vi "Meas Result Generate TWM InpZ Correction - Process Measurement.vi"(7 "table ref":refnum<vi>, 8 "error in":errorcluster, 10 "inpz unc config":T1, 11 "meas":T4={"swp cfg"={"N"=0, "R"=0, "f list"=[], "smpl delay"=0.0, "set delay"=0.0, "set delay np"=0.0, "meas root"=path "", "meas name"="", "meas a-index"=FALSE, "rnd sweep"=FALSE, "mode"=enum."Frequency", "swp mode"=enum."Linear", "avg"=0, "subrec"=0, "multi-freq"=FALSE, "selfcal"=FALSE, "selfcal period [h]"=0.0}, "bridge"={"type"=enum."TWM client", "TWM"={"pipe name"="", "parameters"=[], "handle"=0, "fixed aper [s]"=0.0, "f-list [Hz]"=[], "discrete f-list"=FALSE, "unc mode"=enum."None", "unc mcc"=0, "unc first"=FALSE, "alg id"=enum."TWM-LowZ - Low Z measurement"}, "last f"=0.0, "bias comp"={"bias type"=enum."dummy", "VISA"="", "Enable"=FALSE, "channel qu"=[], "channel Uinit"=[]}, "sim mode"=enum."Generic RLC network", "channel idns"=[], "sim phases"=1}, "src"={"type"=enum."Tektronix AFG3101C", "afg"={"VISA"="", "const"=0.0, "gen DC"=FALSE, "ext ref"=FALSE}, "cDAQ dds"={"device"="", "channels"=[], "mclk source"="", "mclk [Hz]"=0.0, "fs [Hz]"=0.0, "block [s]"=0.0, "buf [s]"=0.0, "task"="", "cmd queue"=refnum, "proc ref"=refnum, "smpl clock out"="/cDAQ3/PFI0", "export smpl clock"=FALSE, "DC ofs [V]"=[], "timebase source"="", "timebase mode"=enum."Local", "dither"=enum."Disabled", "dither level"=0.0, "phase [rad]"=[]}, "gain [V/A]"=1.0, "F5xxx session"={"VISA"="", "mode"=enum."AC voltage", "Earth on"=FALSE, "Ext ref lock"=FALSE}, "t3awg"={"VISA"="", "use ext ref"=FALSE, "ext ref [Hz]"=0.0, "load Z"=enum."High Z", "ramdac max n"=0, "noise dither [V]"=0.0, "t3awg fs rules"=[], "channels"=0, "ramdac min n"=0}}, "results"=refnum, "dvm"={"type"=enum."Disabled", "F5790"={"VISA"="", "Input"=enum."input 1", "Digital filter restart"=enum."medium", "hi resolution"=enum."off", "Digital filter mode"=enum."off", "ext guard"=FALSE}}, "thermo"={"type"=enum."COMET Tx5xx (ethernet)", "comment"="", "tag"="", "refresh"=5.0, "IP"="", "port"=502, "VISA"="", "last readout"=timestamp(0 s since 1904-01-01), "TCP ref"=refnum, "VISA sess"="", "idn"="", "press"=0.0, "RH"=0.0, "temp"=0.0, "pres cor"=[], "RH cor"=[], "temp cor"=[], "try left"=0, "failed"=FALSE, "RTD set"=[], "RTD inv"=[], "range"=0.0, "net mode"=enum."MODBUS", "try fail"=enum."Stop trying - return NaN", "timeout [s]"=0.0, "max retries"=0, "sim t [deg]"=0.0, "status"=0}} {"thermo"."status" items=["ok", "retry", "failed"]; "thermo"."RTD inv" format="%.1f"; "thermo"."RTD set" format="%.1f"; "thermo"."temp cor" format="%.1f"; "thermo"."RH cor" format="%.1f"; "thermo"."pres cor" format="%.1f"; "thermo"."refresh" min=0.1 max=1000.0 format="%.2f"; "src"."t3awg"."t3awg fs rules"."fs-step [Hz]" format="%#_6p"; "src"."t3awg"."t3awg fs rules"."fs-max [Hz]" format="%#_6p"; "src"."t3awg"."t3awg fs rules"."for f0 <" format="%#_6p"; "src"."t3awg"."t3awg fs rules"."fs-min [Hz]" format="%#_6p"; "src"."cDAQ dds"."channels" min=0 step=1; "bridge"."TWM"."f-list [Hz]" format="%#_6p"; "swp cfg"."f list"."bias" format="%#_3p"; "swp cfg"."f list"."level" format="%#_3p"; "swp cfg"."f list"."fs [Hz]" format="%#_5p"; "swp cfg"."f list"."time [s]" format="%#_3p"; "swp cfg"."f list"."f/fs" format="%#_3p"; "swp cfg"."f list"."periods" format="%#_3f"; "swp cfg"."f list"."f [Hz]" format="%#_5p"}) -> (0 "error out":errorcluster, 3 "correction data":T2)   [LabVIEW 2020]
doc: "Generates input impedance correction matrix for TWM."
uses:
  meas session.ctl
  Meas Sweep Config.ctl
  Meas Freq Info.ctl
  meas_swp_mode.ctl
  meas_sweep_flist_mode.ctl
  bridge/Bridge Session.ctl
  bridge/Bridge Type.ctl
  drivers/TWM client/TWM Session.ctl
  drivers/TWM client/TWM parameters.ctl
  drivers/TWM client/Meas Proc QWTB Uncertainty Mode.ctl
  bridge/Bridge Algorithm.ctl
  bridge/Bridge Bias Session.ctl
  bridge/Bridge Bias Type.ctl
  bridge/Bridge Sim Mode.ctl
  source/Source Session.ctl
  source/Source Type.ctl
  drivers/AFG3101C/AFG3101C Session.ctl
  drivers/cDAQ DDS/cDAQ DDS Session.ctl
  drivers/cDAQ DDS/cDAQ DDS Setup.ctl
  drivers/cDAQ DDS/cDAQ DDS Timebase Mode.ctl
  drivers/cDAQ DDS/cDAQ DDS Dither.ctl
  drivers/Fluke 5XXX/top_lev/F5xxx_session.ctl
  drivers/Fluke 5XXX/top_lev/F5xxx_output_mode.ctl
  drivers/T3AWG3K/toplevel/T3AWG Session.ctl
  drivers/T3AWG3K/toplevel/T3AWG Load Z.ctl
  drivers/T3AWG3K/toplevel/fgen_ramdac_fs_rules.ctl
  results/Meas Results Ref.ctl
  results/Meas Results.ctl
  bridge/Bridge Frequency Readings Data.ctl
  drivers/TWM client/Meas Proc QWTB Spectrum Data.ctl
  drivers/TWM client/TWM Phase Info.ctl
  dvm/dvm session.ctl
  dvm/dvm type.ctl
  drivers/Fluke 5790A/top_level/F5790 session.ctl
  thermo/thermo.ctl
  thermo/thermo_types.ctl
  thermo/Thermometer Fail Action.ctl
  Meas Results TWM Digitizer Correction Data.ctl
  results/Meas Results Correction Structuring Mode.ctl
  Meas Results TWM InpZ Correction Uncertainty Config.ctl
  results/Meas Results Sweep Data Uncertainty Mode.ctl
  results/Impedance Equivalent Circuit.ctl
  drivers/T3AWG3K/Active Technologies AWG3000.lvlib
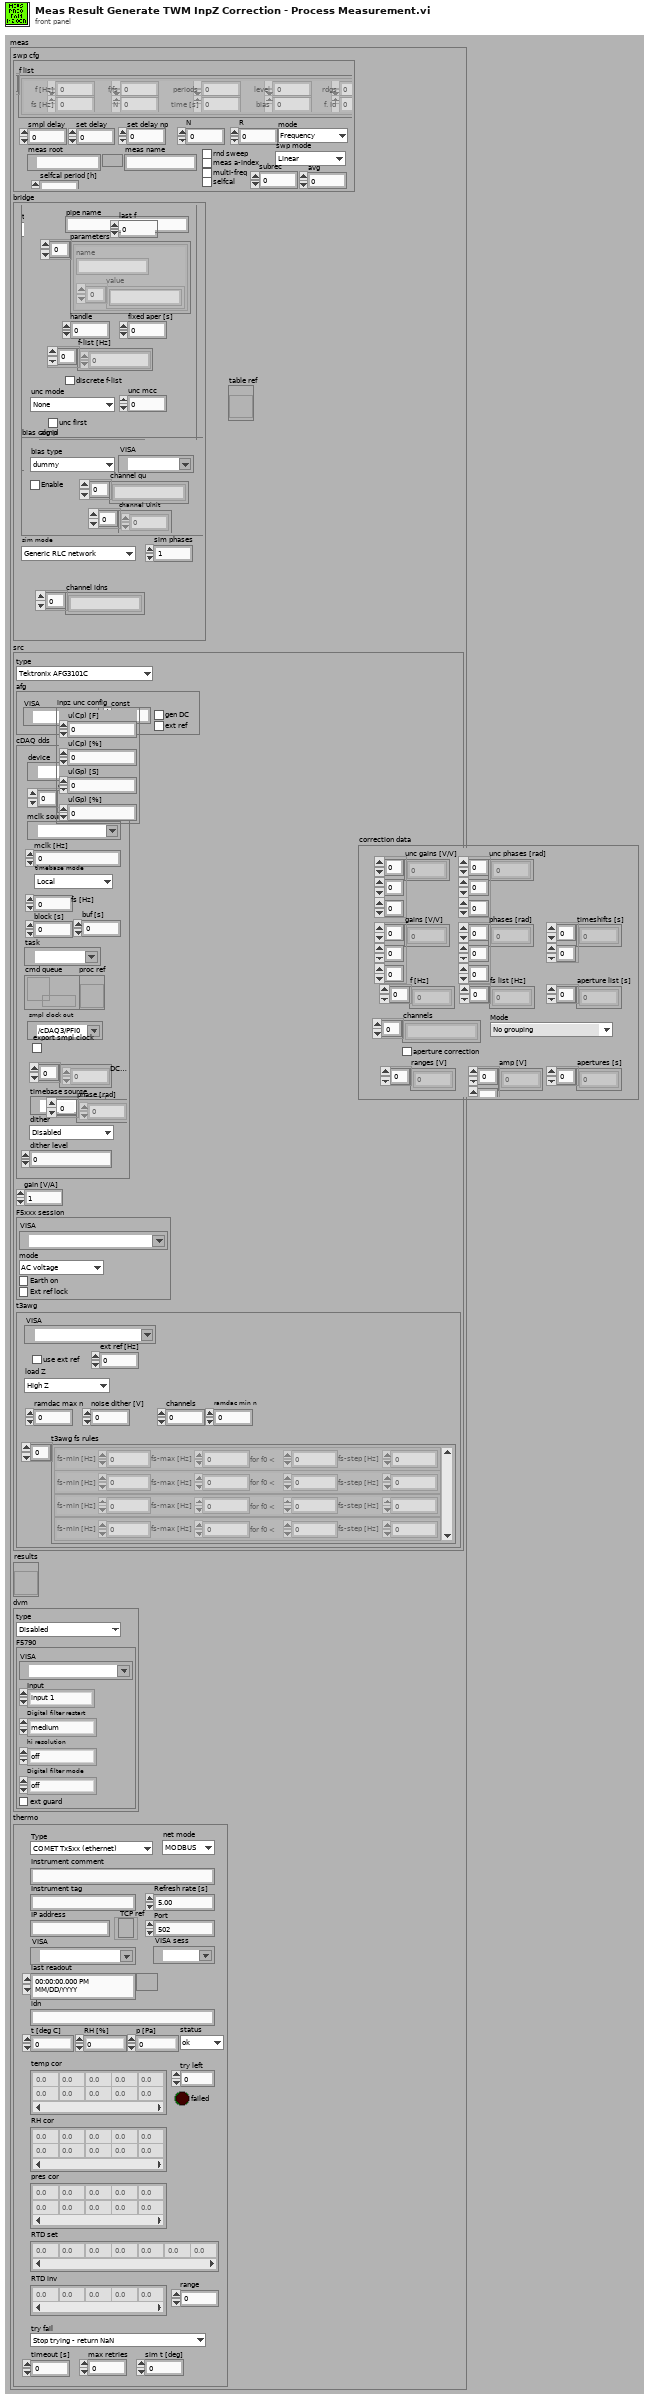
[diagram p1: front panel]
types:
  T1 = typedef "Meas Results TWM InpZ Correction Uncertainty Config.ctl" = cluster{"u(Cp) [F]":dbl, "u(Cp) [%]":dbl, "u(Gp) [S]":dbl, "u(Gp) [%]":dbl}
  T2 = typedef "Meas Results TWM Digitizer Correction Data.ctl" = cluster{"gains [V/V]":dbl[][][], "phases [rad]":dbl[][][], "timeshifts [s]":dbl[][], "f [Hz]":dbl[], "fs list [Hz]":dbl[], "aperture list [s]":dbl[], "channels":string[], "Mode":T3, "aperture correction":bool, "ranges [V]":dbl[], "amp [V]":dbl[][], "apertures [s]":dbl[], "unc gains [V/V]":dbl[][][], "unc phases [rad]":dbl[][][]}
  T3 = typedef "Meas Results Correction Structuring Mode.ctl" = enum16{"No grouping", "Group by apertures (3458A)", "Group by fs (generic digitizer)"}
  T4 = typedef "meas session.ctl" = cluster{"swp cfg":T5, "bridge":T9, "src":T18, "results":T29, "dvm":T30, "thermo":T33}
  T5 = typedef "Meas Sweep Config.ctl" = cluster{"N":i32, "R":i32, "f list":T6[], "smpl delay":dbl, "set delay":dbl, "set delay np":dbl, "meas root":path, "meas name":string, "meas a-index":bool, "rnd sweep":bool, "mode":T7, "swp mode":T8, "avg":i32, "subrec":i32, "multi-freq":bool, "selfcal":bool, "selfcal period [h]":dbl}
  T6 = typedef "Meas Freq Info.ctl" = cluster{"f [Hz]":dbl, "periods":dbl, "f/fs":dbl, "time [s]":dbl, "fs [Hz]":dbl, "N":i32, "level":dbl, "bias":dbl, "rdgs":i32, "f. id":i32}
  T7 = typedef "meas_swp_mode.ctl" = enum16{"Frequency", "Level", "Bias"}
  T8 = typedef "meas_sweep_flist_mode.ctl" = enum16{"Linear", "Log10"}
  T9 = typedef "Bridge Session.ctl" = cluster{"type":T10, "TWM":T11, "last f":dbl, "bias comp":T15, "sim mode":T17, "channel idns":string[], "sim phases":i32}
  T10 = typedef "Bridge Type.ctl" = enum16{"TWM client", "dummy"}
  T11 = typedef "TWM Session.ctl" = cluster{"pipe name":string, "parameters":T12[], "handle":i32, "fixed aper [s]":dbl, "f-list [Hz]":dbl[], "discrete f-list":bool, "unc mode":T13, "unc mcc":i32, "unc first":bool, "alg id":T14}
  T12 = typedef "TWM parameters.ctl" = cluster{"name":string, "value":string[]}
  T13 = typedef "Meas Proc QWTB Uncertainty Mode.ctl" = enum16{"None", "GUF", "Monte Carlo"}
  T14 = typedef "Bridge Algorithm.ctl" = enum16{"TWM-LowZ - Low Z measurement", "TWM-InpZ - Digitizer input Z measurement", "TWM-TIAZ - High Z using TIA"}
  T15 = typedef "Bridge Bias Session.ctl" = cluster{"bias type":T16, "VISA":refnum<visa-resource-name>, "Enable":bool, "channel qu":string[], "channel Uinit":dbl[]}
  T16 = typedef "Bridge Bias Type.ctl" = enum16{"dummy", "CMI LiBbias V1.0"}
  T17 = typedef "Bridge Sim Mode.ctl" = enum16{"Generic RLC network", "Interchannel transfer", "Input impedance"}
  T18 = typedef "Source Session.ctl" = cluster{"type":T19, "afg":T20, "cDAQ dds":T21, "gain [V/A]":dbl, "F5xxx session":T24, "t3awg":T26}
  T19 = typedef "Source Type.ctl" = enum16{"Tektronix AFG3101C", "cDAQ DAC", "Fluke 5xxx", "Agilent 33120A", "R&S SMT", "Teledyne LeCroy T3AWG", "dummy"}
  T20 = typedef "AFG3101C Session.ctl" = cluster{"VISA":refnum<visa-resource-name>, "const":dbl, "gen DC":bool, "ext ref":bool}
  T21 = typedef "cDAQ DDS Session.ctl" = cluster{"device":tag, "channels":i32[], "mclk source":tag, "mclk [Hz]":dbl, "fs [Hz]":dbl, "block [s]":dbl, "buf [s]":dbl, "task":refnum<k21>, "cmd queue":refnum<queue>, "proc ref":refnum<vi>, "smpl clock out":tag, "export smpl clock":bool, "DC ofs [V]":dbl[], "timebase source":tag, "timebase mode":T22, "dither":T23, "dither level":dbl, "phase [rad]":dbl[]}
  T22 = typedef "cDAQ DDS Timebase Mode.ctl" = enum16{"Local", "Take from ADC (e.g. NI 9238)", "Other source"}
  T23 = typedef "cDAQ DDS Dither.ctl" = enum16{"Disabled", "Gaussian"}
  T24 = typedef "F5xxx_session.ctl" = cluster{"VISA":refnum<visa-resource-name>, "mode":T25, "Earth on":bool, "Ext ref lock":bool}
  T25 = typedef "F5xxx_output_mode.ctl" = enum16{"AC voltage", "AC current"}
  T26 = typedef "Active Technologies AWG3000.lvlib/T3AWG Session.ctl" = cluster{"VISA":refnum<visa-resource-name>, "use ext ref":bool, "ext ref [Hz]":dbl, "load Z":T27, "ramdac max n":i32, "noise dither [V]":dbl, "t3awg fs rules":T28[], "channels":i32, "ramdac min n":i32}
  T27 = typedef "Active Technologies AWG3000.lvlib/T3AWG Load Z.ctl" = enum16{"High Z", "50 Ohm"}
  T28 = typedef "Active Technologies AWG3000.lvlib/fgen_ramdac_fs_rules.ctl" = cluster{"fs-min [Hz]":dbl, "fs-max [Hz]":dbl, "for f0 < ":dbl, "fs-step [Hz]":dbl}
  T29 = typedef "Meas Results Ref.ctl" = refnum<vi>
  T30 = typedef "dvm session.ctl" = cluster{"type":T31, "F5790":T32}
  T31 = typedef "dvm type.ctl" = enum16{"Disabled", "Simulated", "Fluke 5790A"}
  T32 = typedef "F5790 session.ctl" = cluster{"VISA":refnum<visa-resource-name>, "Input":enum16{"input 1", "input 2", "wide-band"}, "Digital filter restart":enum16{"medium", "fine", "coarse"}, "hi resolution":enum16{"off", "on"}, "Digital filter mode":enum16{"off", "fast", "medium", "slow"}, "ext guard":bool}
  T33 = typedef "thermo.ctl" = cluster{"type":T34, "comment":string, "tag":string, "refresh":dbl, "IP":string, "port":u16, "VISA":refnum<visa-resource-name>, "last readout":timestamp, "TCP ref":refnum<k5>, "VISA sess":refnum<visa-resource-name>, "idn":string, "press":dbl, "RH":dbl, "temp":dbl, "pres cor":dbl[][], "RH cor":dbl[][], "temp cor":dbl[][], "try left":i32, "failed":bool, "RTD set":dbl[], "RTD inv":dbl[], "range":dbl, "net mode":enum16{"MODBUS", "HTTP"}, "try fail":T35, "timeout [s]":dbl, "max retries":i32, "sim t [deg]":dbl, "status":u16}
  T34 = typedef "thermo_types.ctl" = enum16{"Disabled", "Simulated", "COMET Tx5xx (ethernet)", "Keithley 2002 (GPIB) + RTD", "Agilent 344xx (GPIB) + RTD"}
  T35 = typedef "Thermometer Fail Action.ctl" = enum16{"Stop trying - keep last value", "Stop trying - return NaN", "Generate error - stop sweep"}
  T36 = typedef "Meas Results Sweep Data Uncertainty Mode.ctl" = enum16{"ua(y)", "ua(y) (p=95%)", "uc(y) (p=95%)"}
  T37 = typedef "Meas Results.ctl" = cluster{"freqs":T38[][], "locked":bool, "last fid":i32, "modified":bool, "mjr name":string, "mnr name":string, "last spectra":T39[][], "saved?":bool, "TWM phase":T40[], "time start":timestamp, "time stop":timestamp, "equ cct":string}
  T38 = typedef "Bridge Frequency Readings Data.ctl" = cluster{"Udut":dbl[], "Iref":dbl[], "Udc":dbl[], "Idc":dbl[], "mjr":dbl[], "mnr":dbl[], "mjr_sh":dbl[], "mnr_sh":dbl[], "u(mjr)":dbl[], "u(mnr)":dbl[], "ua2(mjr)":dbl[], "ua2(mnr)":dbl[], "n":i32, "f [Hz]":dbl, "fs [Hz]":dbl, "aperture [s]":dbl, "Udvm":dbl[], "u(Udvm) [V]":dbl, "t_dut [degC]":dbl[], "RH_dut [%]":dbl[], "p_dut [Pa]":dbl[], "timestamp":timestamp[]}
  T39 = typedef "Meas Proc QWTB Spectrum Data.ctl" = cluster{"x":sgl[], "y":sgl[], "label":string}
  T40 = typedef "TWM Phase Info.ctl" = cluster{"ref chn id (I)":string, "dut chn id (U)":string, "ref chn range [V]":dbl, "dut chn range [V]":dbl, "aperture [s]":dbl, "fs [Hz]":dbl, "ref chn transducer (I)":string, "dut chn transducer (U)":string}
  T41 = typedef "Impedance Equivalent Circuit.ctl" = enum16{"Keep original", "Rs-Xs", "Gp-Bp", "Z-phid", "Z-phir", "Y-phid", "Y-phir", "Cp-D", "Cp-Q", "Cp-Rp", "Cp-Gp", "Cs-D", "Cs-Q", "Cs-Rs", "Ls-Rs", "Ls-Q", "Rs-Tau"}
  T42 = typedef "Meas Results Sweep Data.ctl" = cluster{"Udut":dbl[], "Iref":dbl[], "Udc":dbl[], "Idc":dbl[], "mjr":dbl[], "mnr":dbl[], "mjr_sh":dbl[], "mnr_sh":dbl[], "f [Hz]":dbl[], "n [-]":i32[], "fs [Hz]":dbl[], "aperture [s]":dbl[], "Udvm":dbl[], "t_dut [degC]":dbl[], "RH_dut [%]":dbl[], "p_dut [Pa]":dbl[]}
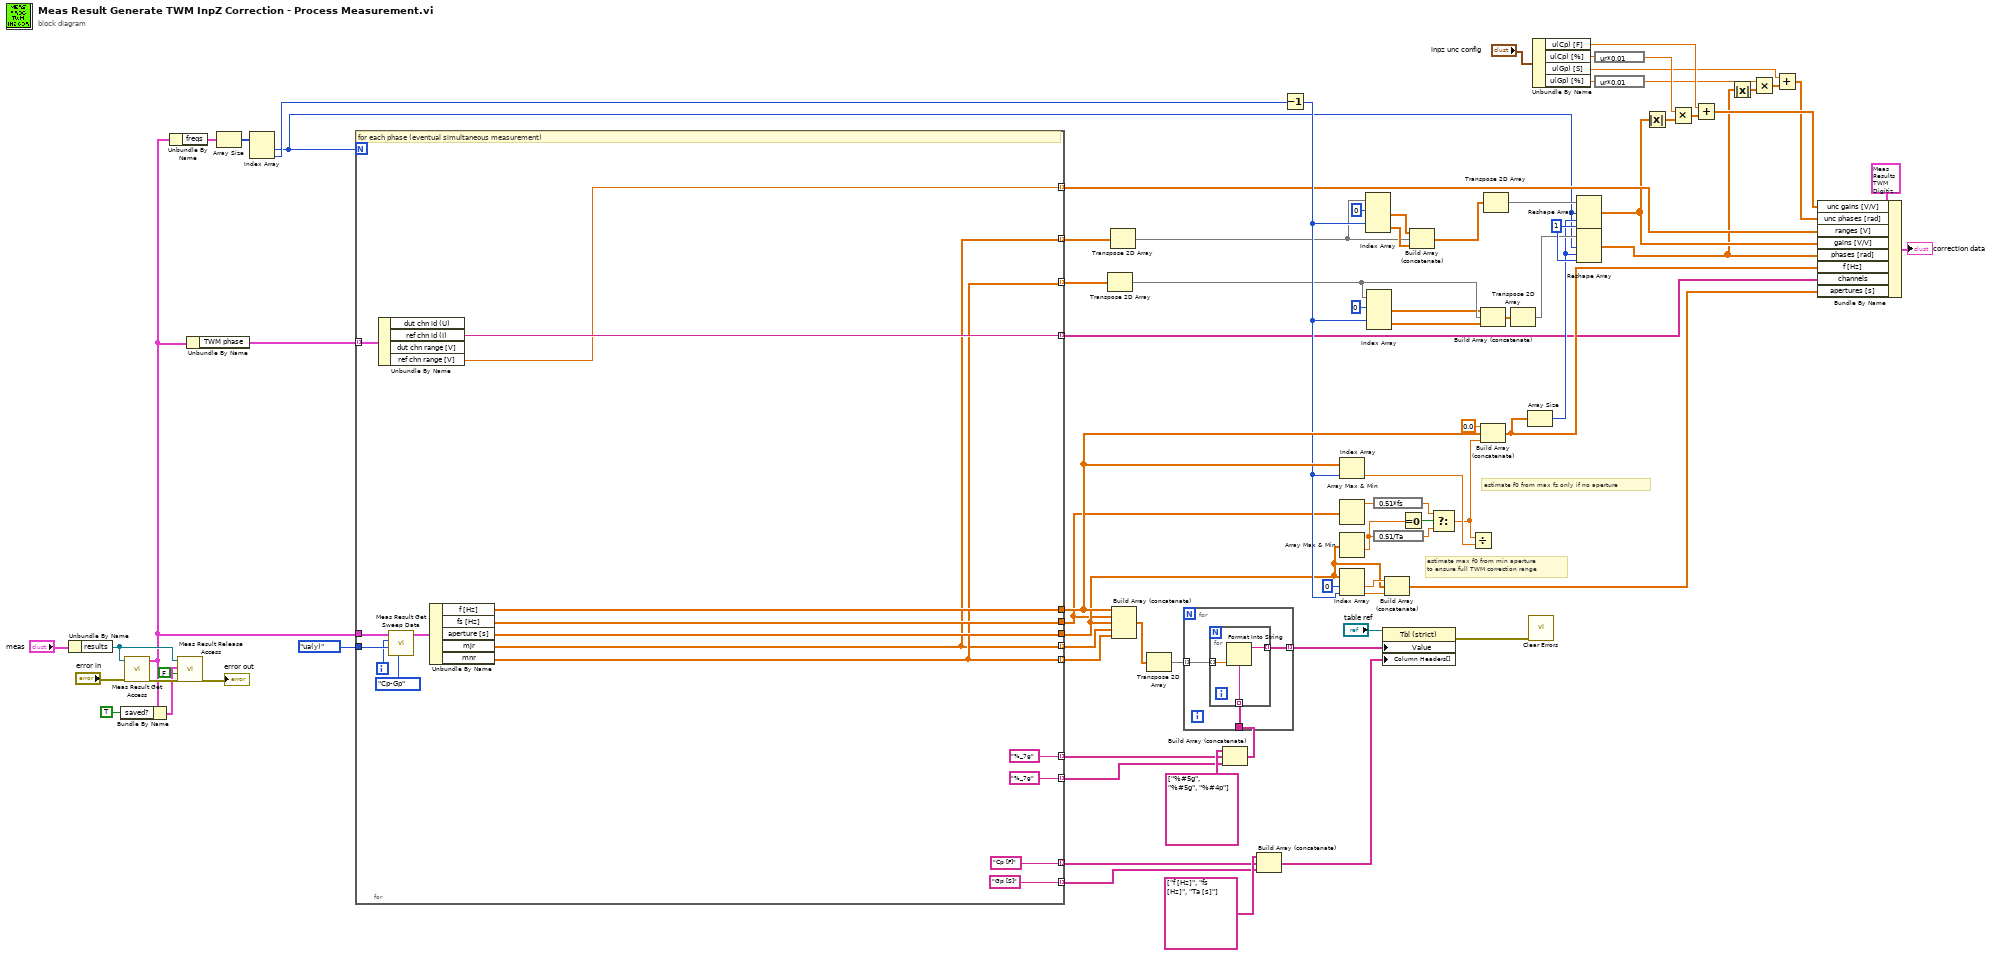
[diagram p0: block diagram]
diagram:
  w38 = 1 ("dimension size")
  # "estimate f0 from max fs only if no aperture"
  # "estimate max f0 from min aperture\nto ensure full TWM correction range"
  n1 = Unbundle By Name("meas") -> ("results"=w76:T29)
  n2 = call "Meas Result Get Access.vi"("error in"="error in", "results ref"=w76) -> ("error out"=w79:errorcluster, "results data"=w64:T37)  [unwired: 8 in]
  n3 = Bundle By Name(cluster=w64, "saved?"=TRUE) -> (w77:T37)
  n4 = Unbundle By Name(w64) -> ("freqs"=w81:T38[][])
  n5 = call "Meas Result Release Access.vi"("error in"=w79, "Release only (True)"=FALSE, "results data in"=w77, "results ref"=w76) -> ("error out"=→"error out":errorcluster)  [unwired: 7 in]
  n6 = Unbundle By Name(w64) -> ("TWM phase"=w63:T40[])
  n7 = Array Size(array=w81) -> (size(s)=w80:i32[])
  n8 = Index Array(array=w80) -> (element #1=w28:i32, element #2=w39:i32)  [unwired: 2 in]
  n9 = for {
    N: w28 -> [_]
    tunnel: Meas_Results_Sweep_Data_Uncertainty_Mode."ua(y)" ("uncertainty mode") -> [w98]
    tunnel: w64 -> [w92]
    tunnel: [w97] -> w55
    tunnel: [w96] -> w7
    tunnel: [w95] -> w8
    tunnel: [w85] -> w70 mode=indexing
    tunnel: [w86] -> w69 mode=indexing
    tunnel: ["%_7g"] -> w67 mode=indexing
    tunnel: ["%_7g"] -> w66 mode=indexing
    tunnel: w63 -> [w91] mode=indexing
    tunnel: ["Cp [F]"] -> w52 mode=indexing
    tunnel: ["Gp [S]"] -> w51 mode=indexing
    tunnel: [w87] -> w32 mode=indexing
    tunnel: [w86] -> w31 mode=indexing
    tunnel: [w85] -> w30 mode=indexing
    tunnel: [w84] -> w29 mode=indexing
    i -> [w90]
    # "for each phase (eventual simultaneous measurement)"
    n10 = Unbundle By Name(w91) -> ("ref chn id (I)"=w87:string, "ref chn range [V]"=w84:dbl)  [unwired: 2 out]
    n11 = call "Meas Result Get Sweep Data.vi"("equ connection override"=Impedance_Equivalent_Circuit."Cp-Gp", "uncertainty mode"=w98, "phase index (default: 0)"=w90, "result"=w92) -> ("data"=w99:T42)  [unwired: 5 in, 2 out]
    n12 = Unbundle By Name(w99) -> ("f [Hz]"=w97:dbl[], "fs [Hz]"=w96:dbl[], "aperture [s]"=w95:dbl[], "mjr"=w85:dbl[], "mnr"=w86:dbl[])
  }
  n13 = Transpose 2D Array(2D array=w31) -> (transposed array=w26:dbl[][])
  n14 = Transpose 2D Array(2D array=w30) -> (transposed array=w27:dbl[][])
  n15 = Build Array (concatenate)(w55, w7, w8, w70, w69) -> (w71:dbl[][])
  n16 = Transpose 2D Array(2D array=w71) -> (transposed array=w72:dbl[][])
  n17 = Build Array (concatenate)(string[] ["%#5g", "%#5g", "%#4p"], w67, w66) -> (w65:string[])
  n18 = for {
    tunnel: w72 -> [w101] mode=indexing
    tunnel: w65 -> [w102]
    tunnel: [w100] -> w49 mode=indexing
    n19 = for {
      tunnel: w102 -> [w104] mode=indexing
      tunnel: w101 -> [w105] mode=indexing
      tunnel: [w103] -> w100 mode=indexing
      n20 = Format Into String(format string=w104, w105) -> (resulting string=w103:string)  [unwired: 2 in, 1 out]
    }
  }
  n21 = Build Array (concatenate)(string[] ["f [Hz]", "fs [Hz]", "Ta [s]"], w52, w51) -> (w48:string[])
  n22 = Decrement(x=w39) -> (x-1=w40:i32)
  n23 = Index Array(array=w55, index=w40) -> (element=w57:dbl)
  n24 = Array Max & Min(array=w7) -> (max value=w1:dbl)  [unwired: 3 out]
  n25 = Array Max & Min(array=w8) -> (min value=w6:dbl)  [unwired: 3 out]
  n26 = Index Array(array=w8, index #1=0 ("index"), index #2=w40) -> (element #1=w45:dbl, element #2=w44:dbl)
  n27 = Index Array(array=w27, index (row) #1=0 ("index (row)"), index (row) #2=w40) -> (element #1=w60:dbl[], element #2=w59:dbl[])  [unwired: 2 in]
  n28 = Index Array(array=w26, index (row) #1=0 ("index (row)"), index (row) #2=w40) -> (element #1=w25:dbl[], element #2=w24:dbl[])  [unwired: 2 in]
  n29 = expression code="0.51*fs"(w1) -> (w4:dbl)
  n30 = expression code="0.51/Ta"(w6) -> (w3:dbl)
  n31 = property class="Tbl (strict)"(reference="table ref", "Value"=w49, "Column Headers[]"=w48) -> (error out=w47:errorcluster)  [unwired: 1 in, 1 out]
  n32 = Build Array (concatenate)(w45, w8, w44) -> (w43:dbl[])
  n33 = Equal To 0?(x=w6) -> (x = 0?=w5:bool)
  n34 = Build Array (concatenate)(w60, w27, w59) -> (w42:dbl[][])
  n35 = Select(t=w4, s=w5, f=w3) -> (s? t:f=w2:dbl)
  n36 = Divide(x=w2, y=w57) -> ()  [unwired: 1 out]
  n37 = Build Array (concatenate)(w25, w26, w24) -> (w41:dbl[][])
  n38 = Build Array (concatenate)(0.0 ("element"), w55, w2) -> (w35:dbl[])
  n39 = Transpose 2D Array(2D array=w42) -> (transposed array=w36:dbl[][])
  n40 = Transpose 2D Array(2D array=w41) -> (transposed array=w37:dbl[][])
  n41 = Array Size(array=w35) -> (size(s)=w34:i32)
  n42 = call <vilib>:"Clear Errors.vi"("error in (no error)"=w47) -> ()  [unwired: 5 in, 2 out]
  n43 = Unbundle By Name("inpz unc config") -> ("u(Cp) [F]"=w18:dbl, "u(Cp) [%]"=w22:dbl, "u(Gp) [S]"=w11:dbl, "u(Gp) [%]"=w16:dbl)
  n44 = Reshape Array(w36, w28, w34, w38) -> (w20:dbl[][][])
  n45 = Reshape Array(w37, w28, w34, w38) -> (w13:dbl[][][])
  n46 = expression code="ur*0.01"(w22) -> (w21:dbl)
  n47 = expression code="ur*0.01"(w16) -> (w14:dbl)
  n48 = Absolute Value(x=w20) -> (abs(x)=w9:dbl[][][])
  n49 = Multiply(x=w21, y=w9) -> (x*y=w19:dbl[][][])
  n50 = Add(x=w18, y=w19) -> (x+y=w17:dbl[][][])
  n51 = Absolute Value(x=w13) -> (abs(x)=w10:dbl[][][])
  n52 = Multiply(x=w14, y=w10) -> (x*y=w15:dbl[][][])
  n53 = Add(x=w11, y=w15) -> (x+y=w12:dbl[][][])
  n54 = Bundle By Name(cluster=T2 {"gains [V/V]"=[], "phases [rad]"=[], "timeshifts [s]"=[], "f [Hz]"=[], "fs list [Hz]"=[], "aperture list [s]"=[], "channels"=[], "Mode"=enum."No grouping", "aperture correction"=FALSE, "ranges [V]"=[], "amp [V]"=[], "apertures [s]"=[], "unc gains [V/V]"=[], "unc phases [rad]"=[]} ("correction data"), "unc gains [V/V]"=w17, "unc phases [rad]"=w12, "ranges [V]"=w29, "gains [V/V]"=w20, "phases [rad]"=w13, "f [Hz]"=w35, "channels"=w32, "apertures [s]"=w43) -> (→"correction data":T2)
